vi "Set_algorithm.vi"(8 "error in (no error)":errorcluster, 10 "Appliance.lvclass":refnum<class "Appliance.lvclass">, 11 "Chef in":refnum<class "Chef.lvclass">) -> (0 "error out":errorcluster, 3 "Chef out":refnum<class "Chef.lvclass">)   [LabVIEW 2020, in "Chef.lvclass"]
uses:
  Chef.lvclass
  Appliance/Appliance.lvclass
  Chef.lvclass/Chef.ctl
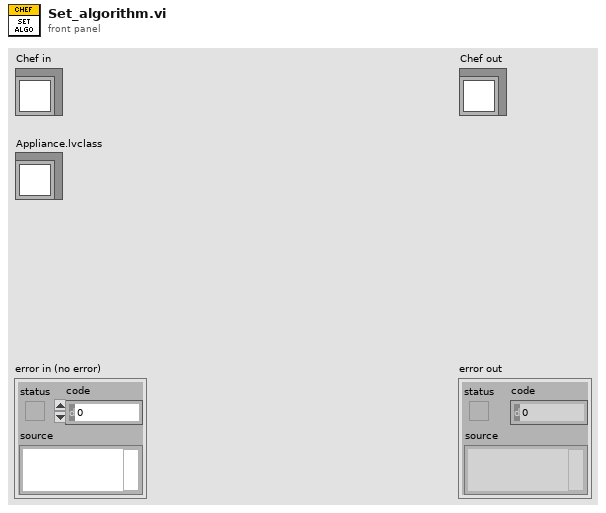
[diagram p1: front panel]
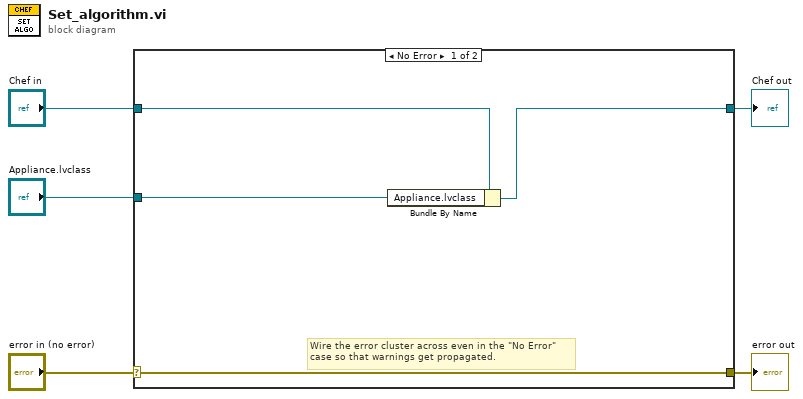
[diagram p0: block diagram]
diagram:
  n1 = case shown="No Error" "error in (no error)" {
    selector: "error in (no error)" -> [w9 w11]
    tunnel: [w9 w11] -> w4
    tunnel: [w6 w10] -> w2
    tunnel: "Chef in" -> [w8 w10]
    tunnel: "Appliance.lvclass" -> [w7 _]
    frame No Error {
      # "Wire the error cluster across even in the \"No Error\"\ncase so that warnings get propagated."
      n2 = Bundle By Name(cluster=w8, "Appliance.lvclass"=w7) -> (w6:refnum<class "Chef.lvclass">)
    }
    frame Error {
    }
  }
  "error out" <- w4
  "Chef out" <- w2
